vi "Distribute.vi"(8 "error in (no error)":errorcluster, 10 "Bounds":T1, 11 "Container in":refnum<class "IContainer.lvclass">) -> (0 "error out":errorcluster, 2 "Bounds":T1[](array[typedef]), 3 "Container out":refnum<class "IContainer.lvclass">, 5 "Visible bounds":T1[](array[typedef]), 7 "Visible indices":i32[](array[numeric]))   [LabVIEW 2021, in "IContainer.lvclass"]
doc: "Copyright 2018, Wiebe Walstra, wiebe@carya.nl."
uses:
  IContainer.lvclass
  <vilib>/Utility/miscctls.llb/LVRectTypeDef.ctl
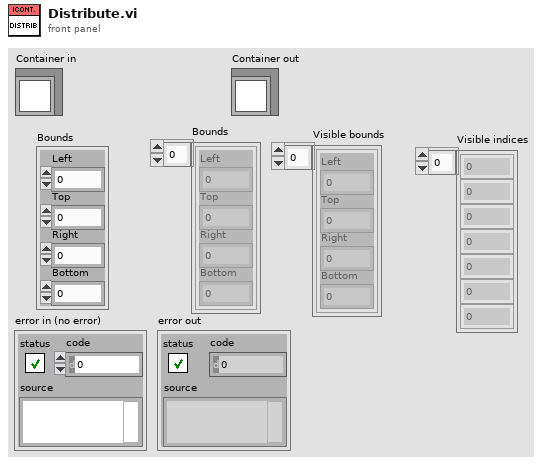
[diagram p1: front panel]
types:
  T1 = typedef "LVRectTypeDef.ctl" = cluster{"Left":i16, "Top":i16, "Right":i16, "Bottom":i16}
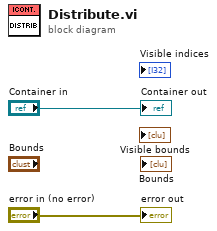
[diagram p0: block diagram]
diagram:
  "error out" <- "error in (no error)"
  "Container out" <- "Container in"
